vi "BypassAndLogErrors.vi"(7 "Bypass Errors":bool, 8 "error in (no error)":errorcluster, 11 "Log File Path":path) -> (0 "error out":errorcluster)   [LabVIEW 2015]
panel:
  out "resulting string":string
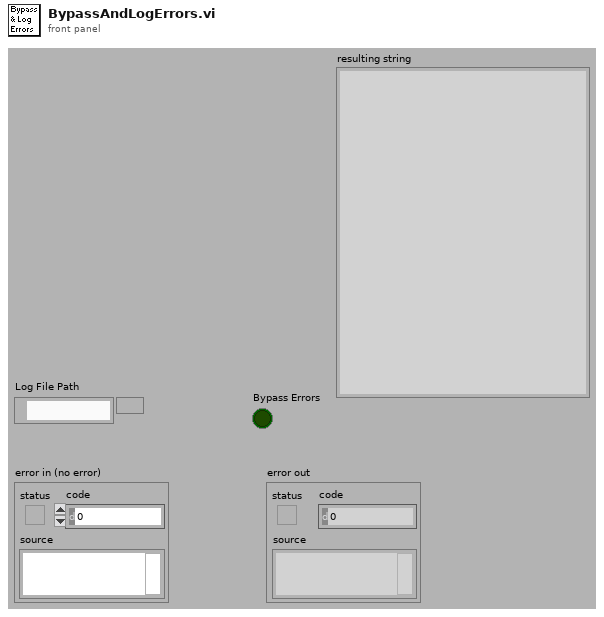
[diagram p1: front panel]
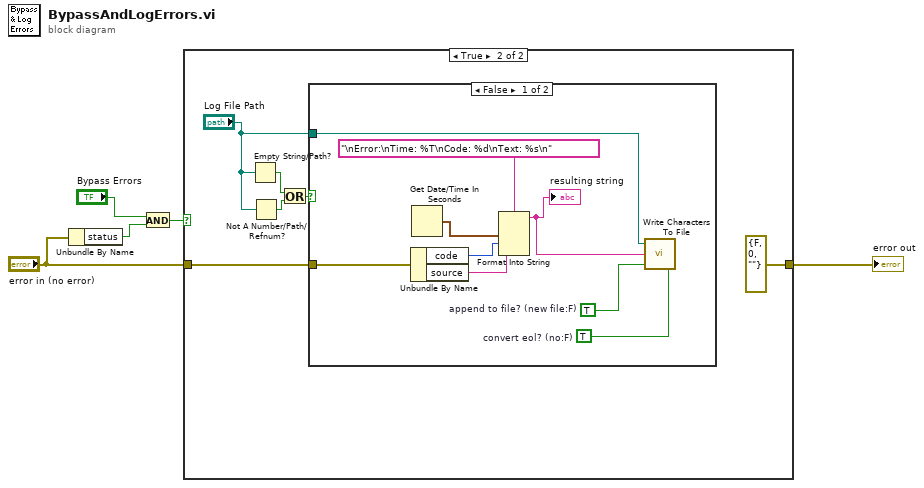
[diagram p0: block diagram]
diagram:
  n1 = Unbundle By Name("error in (no error)") -> ("status"=w2:bool)
  n2 = And(x="Bypass Errors", y=w2) -> (x .and. y?=w1:bool)
  n3 = case shown="True" w1 {
    tunnel: [w6 errorcluster {"status"=FALSE, "code"=0, "source"=""} ("error in (no error)")] -> w5
    tunnel: "error in (no error)" -> [w6 w11]
    frame False {
    }
    frame True {
      n4 = Empty String/Path?(string/path="Log File Path") -> (empty?=w8:bool)
      n5 = Not A Number/Path/Refnum?(number/path/refnum="Log File Path") -> (NaN/Path/Refnum?=w9:bool)
      n6 = Or(x=w8, y=w9) -> (x .or. y?=w7:bool)
      n7 = case shown="False" w7 {
        tunnel: w11 -> [w20 _]
        tunnel: "Log File Path" -> [w15 _]
        frame False {
          w13 = TRUE  # convert eol? (no:F)
          w21 = TRUE  # append to file? (new file:F)
          n8 = Unbundle By Name(w20) -> ("code"=w18:i32, "source"=w17:string)
          n9 = Get Date/Time In Seconds() -> (seconds since 1Jan1904=w19:timestamp)
          n10 = Format Into String(format string="\nError:\nTime: %T\nCode: %d\nText: %s\n", w19, w18, w17) -> (resulting string=w16:string)  [unwired: 2 in, 1 out]
          "resulting string" <- w16
          n11 = call <vilib>:"Write Characters To File.vi"("convert eol? (no:F)"=w13, "append to file? (new file:F)"=w21, "character string"=w16, "file path (dialog if empty)"=w15) -> ()  [unwired: 2 out]
        }
        frame True {
        }
      }
    }
  }
  "error out" <- w5
